vi "LVObject to JSON - Base Class - Returns Type.vi"() -> ()   [LabVIEW 2017, in "Tests.lvlib" / "Type Name Handling.lvlib"]
uses:
  Weather Forecast/Weather Forecast.lvclass
  Flatten To JSON Object/Flatten To JSON Object.lvclass
  Flatten To JSON Object/Type Name Handling.ctl
  Flatten To JSON Object/Flatten To JSON Object.lvclass/Flatten To JSON Object.ctl
  Flatten To JSON Object/Write Type Name Handling.vi
  <vilib>/addons/_JKI Toolkits/Caraya/classes/Assert/Assert Equal Value_Variant.vi
  Type Name Handling.lvlib
  <vilib>/addons/_JKI Toolkits/Caraya/classes/Test/Test.lvclass
  <vilib>/addons/_JKI Toolkits/Caraya/classes/Assert/Assert.lvclass
panel:
  out "error out":errorcluster
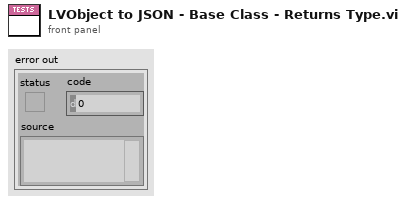
[diagram p1: front panel]
types:
  T1 = typedef "Flatten To JSON Object.lvclass/Type Name Handling.ctl" = enum16{"None", "Inline"}
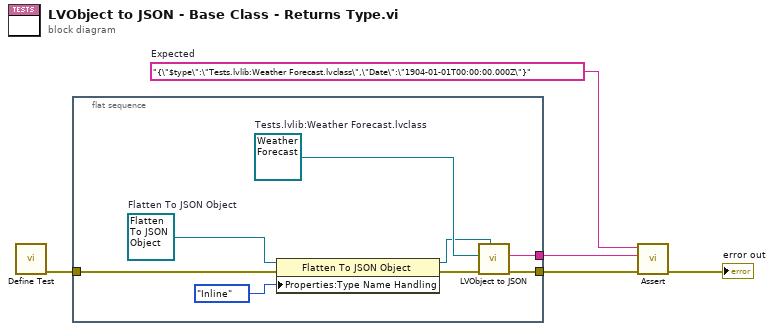
[diagram p0: block diagram]
diagram:
  w2 = "{\"$type\":\"Tests.lvlib:Weather Forecast.lvclass\",\"Date\":\"1904-01-01T00:00:00.000Z\"}"  # Expected
  n1 = call <vilib>:"Define Test.vi"() -> ("error out"=w5:errorcluster)  [unwired: 11 in]
  n2 = flat-sequence {
    tunnel: w5 -> [w7]
    tunnel: [w13] -> w4
    tunnel: [w11] -> w3
    frame #0 {
      w10 = refnum<class "Flatten To JSON Object.lvclass"> refnum  # Flatten To JSON Object
      w12 = refnum<class "Weather Forecast.lvclass"> refnum  # Tests.lvlib:Weather Forecast.lvclass
      n3 = property class="Flatten To JSON Object"(reference=w10, error in=w7, "Properties:Type Name Handling"=Type_Name_Handling."Inline" ("Type Name Handling")) -> (reference out=w9:refnum<class "Flatten To JSON Object.lvclass">, error out=w6:errorcluster)
      n4 = call-dynamic "LVObject to JSON.vi"("Flatten To JSON Object in"=w9, "error in (no error)"=w6, "Object"=w12) -> ("error out"=w13:errorcluster, "<JSON>Object"=w11:string)  [unwired: 7 in]
    }
  }
  n5 = call-poly <vilib>:"Assert.vi"("error in (no error)"=w4, "Y"=w3, "X"=w2) -> ("error out"=→"error out":errorcluster)  [unwired: 8 in]
